vi "Run TS Panel.vi"(8 "error in":errorcluster, 11 "Heat Flow Test Stand in":refnum<class "Heat Flow Test Stand.lvclass">) -> (0 "error out":errorcluster, 3 "Heat Flow Test Stand in":refnum<class "Heat Flow Test Stand.lvclass">)   [LabVIEW 2019, in "Test Stands.lvlib" / "Heat Flow Test Stand.lvclass"]
uses:
  Heat Flow Test Stand.lvclass
  C:/Users/wg/Documents/LV_Projects/test-stand/App/Generic Test Stand/Generic Test Stand.lvclass
  Generic Test Stand/Generic Test Stand.lvclass/Generic Test Stand.ctl
  <vilib>/Utility/error.llb/Error Cluster From Error Code.vi
  <vilib>/ErrorRing/Error Ring.xnode
  Generic Test Stand/Generic Test Stand.lvclass
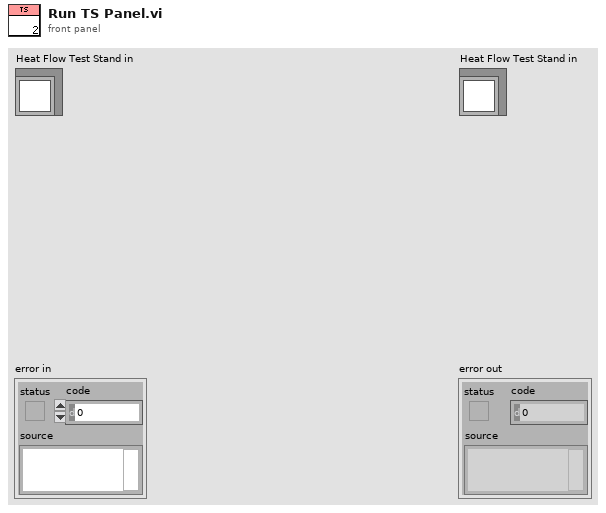
[diagram p1: front panel]
types:
  T1 = enum32{"invalid VI type", "Standard VI", "Control VI", "Global VI", "Polymorphic VI", "Configuration VI", "SubSystem", "Facade VI", "Method VI", "Statechart Diagram VI"}
  T2 = enum32{"Bad", "Idle", "Run top level", "Running"}
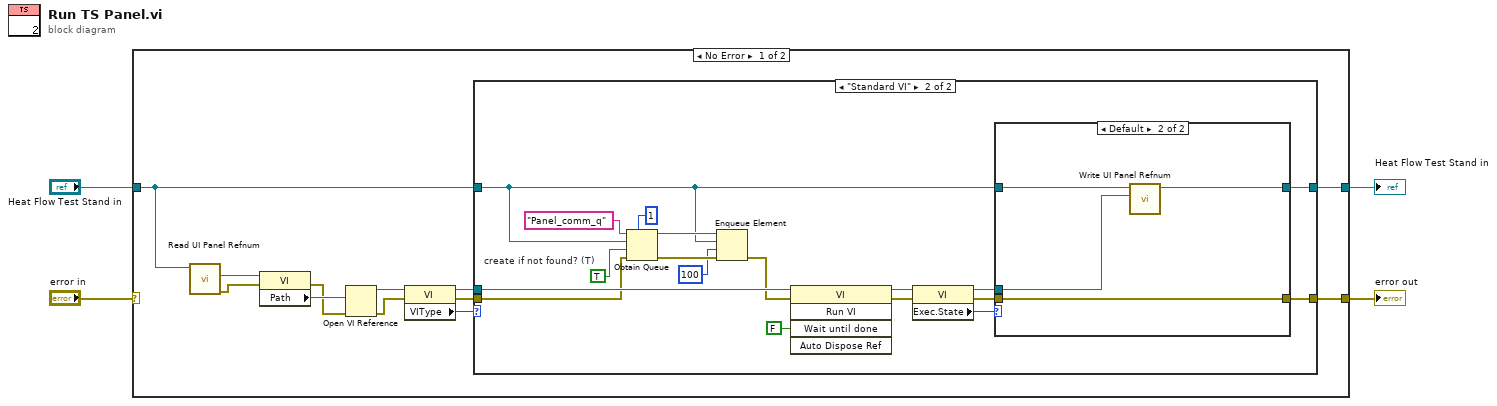
[diagram p0: block diagram]
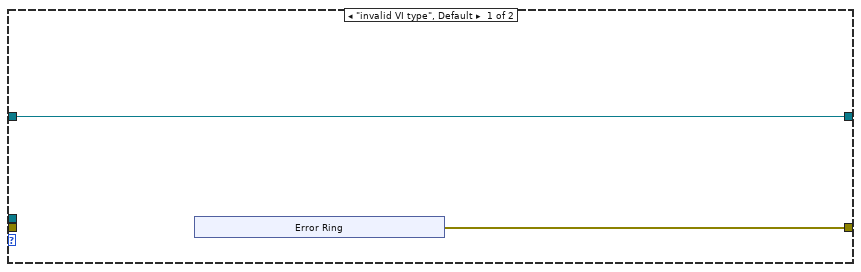
[diagram p2: hidden frame]
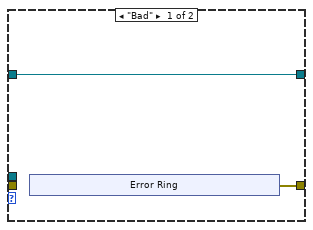
[diagram p3: hidden frame]
diagram:
  n1 = case shown="No Error" "error in" {
    selector: "error in" -> [_ w52]
    tunnel: [w5 w52] -> w2
    tunnel: [w6 w51] -> w1
    tunnel: "Heat Flow Test Stand in" -> [w7 w51]
    frame No Error {
      n2 = call "Read UI Panel Refnum.vi"("Generic Test Stand in"=w7) -> ("error out"=w12:errorcluster, "UI Panel Refnum"=w14:refnum<vi>)  [unwired: 8 in, 1 out]
      n3 = property class="VI"(reference=w14, error in=w12) -> (error out=w11:errorcluster, "Path"=w16:path)  [unwired: 1 out]
      n4 = Open VI Reference(vi path=w16, error in (no error)=w11) -> (vi reference=w15:refnum<vi>, error out=w10:errorcluster)  [unwired: 4 in]
      n5 = property class="VI"(reference=w15, error in=w10) -> (reference out=w13:refnum<vi>, error out=w9:errorcluster, "VIType"=w8:T1)
      n6 = case shown="\"Standard VI\"" w8 {
        tunnel: w13 -> [_ w34]
        tunnel: w9 -> [_ w28]
        tunnel: w7 -> [w18 w26]
        tunnel: [w18 w33] -> w6
        tunnel: [w17 w32] -> w5
        frame "invalid VI type", Default {
          n7 = xnode "Error Ring"() -> ("error out"=w17:errorcluster)
        }
        frame "Standard VI" {
          w29 = TRUE  # create if not found? (T)
          n8 = Obtain Queue(max queue size (-1, unlimited)=1, name (unnamed)="Panel_comm_q", element data type=w26, create if not found? (T)=w29, error in (no error)=w28) -> (queue out=w27:refnum<queue>, error out=w25:errorcluster)  [unwired: 1 out]
          n9 = Enqueue Element(queue=w27, element=w26, timeout in ms (-1)=100, error in (no error)=w25) -> (error out=w23:errorcluster)  [unwired: 2 out]
          n10 = invoke class="VI" method="Run VI"(reference=w34, error in=w23, "Wait until done"=FALSE ("Wait Until Done")) -> (reference out=w37:refnum<vi>, error out=w36:errorcluster)  [unwired: 2 in, 3 out]
          n11 = property class="VI"(reference=w37, error in=w36) -> (reference out=w39:refnum<vi>, error out=w38:errorcluster, "Exec.State"=w40:T2)
          n12 = case shown="Default" w40 {
            tunnel: w39 -> [_ w47]
            tunnel: w38 -> [_ w50]
            tunnel: [w42 w50] -> w32
            tunnel: w26 -> [w41 w49]
            tunnel: [w41 w48] -> w33
            frame "Bad" {
              n13 = xnode "Error Ring"() -> ("error out"=w42:errorcluster)
            }
            frame Default {
              n14 = call "Write UI Panel Refnum.vi"("UI Panel Refnum"=w47, "Generic Test Stand in"=w49) -> ("Generic Test Stand out"=w48:refnum<class "Heat Flow Test Stand.lvclass">)  [unwired: 8 in, 1 out]
            }
          }
        }
      }
    }
    frame Error {
    }
  }
  "error out" <- w2
  "Heat Flow Test Stand in" <- w1
